vi "AbortSingle.vi"(8 "error in (no error)":errorcluster, 9 "taskId":i32(ring) items=["TLibrary", "T01", "T02", "T03", "T04", "T05", "T06", "T07", "T08", "T09", "T10", "T11", "T12", "T13", "T14", "T15", "T16", "T17", "T18", "T19", "T20", "T21", "T22", "T23", "T24", "T25", "T26", "T27", "T28", "T29", "T30", "T31"], 10 "axis name? (all)":string, 11 "controller in":refnum<k24>) -> (0 "error out":errorcluster, 3 "controller out":refnum<k24>)   [LabVIEW 2016, in "Aerotech VIs.lvlib"]
uses:
  Aerotech VIs.lvlib
  C:/Program Files (x86)/Aerotech/A3200/LabVIEW/2010/Bin/Aerotech.A3200.dll
  C:/Program Files (x86)/Aerotech/A3200/LabVIEW/2010/Bin/Aerotech.A3200.LabVIEW.dll
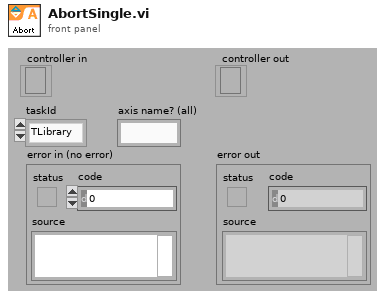
[diagram p1: front panel]
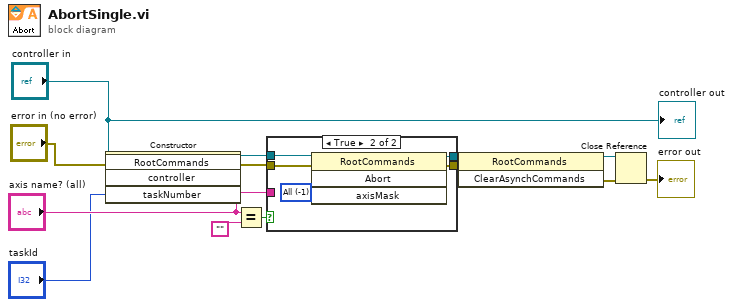
[diagram p0: block diagram]
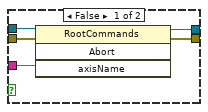
[diagram p2: hidden frame]
diagram:
  n1 = constructor class="RootCommands"(error in="error in (no error)", "controller"="controller in", "taskNumber"="taskId") -> (reference out=w4:refnum<k24>, error out=w2:errorcluster)  [unwired: 2 in, 3 out]
  n2 = Equal?(x="axis name? (all)", y="") -> (x = y?=w11:bool)
  n3 = case shown="True" w11 {
    tunnel: w4 -> [w18 w23]
    tunnel: "axis name? (all)" -> [w14 _]
    tunnel: [w17 w21] -> w6
    tunnel: w2 -> [w16 w22]
    tunnel: [w15 w20] -> w3
    frame False {
      n4 = invoke class="RootCommands" method="Abort"(reference=w18, error in=w16, "axisName"=w14) -> (reference out=w15:refnum<k24>, error out=w17:errorcluster)  [unwired: 1 in, 2 out]
    }
    frame True {
      w19 = -1 items=["None"=0, "A00"=1, "A01"=2, "A02"=4, "A03"=8, "A04"=16, "A05"=32, "A06"=64, "A07"=128, "A08"=256, "A09"=512, "A10"=1024, "A11"=2048, "A12"=4096, "A13"=8192, "A14"=16384, "A15"=32768, "A16"=65536, "A17"=131072, "A18"=262144, "A19"=524288, "A20"=1048576, "A21"=2097152, "A22"=4194304, "A23"=8388608, "A24"=16777216, "A25"=33554432, "A26"=67108864, "A27"=134217728, "A28"=268435456, "A29"=536870912, "A30"=1073741824, "A31"=-2147483648, "All"=-1] ("axisMask")
      n5 = invoke class="RootCommands" method="Abort"(reference=w23, error in=w22, "axisMask"=w19) -> (reference out=w20:refnum<k24>, error out=w21:errorcluster)  [unwired: 1 in, 2 out]
    }
  }
  n6 = invoke class="RootCommands" method="ClearAsynchCommands"(reference=w3, error in=w6) -> (reference out=w9:refnum<k24>, error out=w10:errorcluster)  [unwired: 1 in, 1 out]
  n7 = Close Reference(reference=w9, error in (no error)=w10) -> (error out=→"error out":errorcluster)
  "controller out" <- "controller in"
